vi "Even Number Check.vi"(1 "Number to Test":i32) -> (0 "Even":bool)   [LabVIEW 2014, in "Initialization and IO Node Scripting.lvlib"]
uses:
  Initialization and IO Node Scripting.lvlib
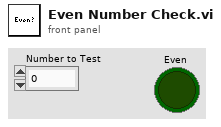
[diagram p1: front panel]
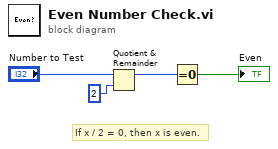
[diagram p0: block diagram]
diagram:
  # "If x / 2 = 0, then x is even."
  n1 = Quotient & Remainder(x="Number to Test", y=2) -> (x-y*floor(x/y)=w2:i32)  [unwired: 1 out]
  n2 = Equal To 0?(x=w2) -> (x = 0?=→"Even":bool)
